vi "Open File for Writing.vi"(8 "error in (no error)":errorcluster, 11 "Configuration File in":refnum<class "Configuration File.lvclass">) -> (0 "error out":errorcluster, 1 "File was Open?":bool, 2 "refnum out":T1, 3 "Configuration File out":refnum<class "Configuration File.lvclass">)   [LabVIEW 2020, in "Configuration File.lvclass"]
doc: "The purpose of this VI is to prevent race conditions when references to files are opened in from many locations."
uses:
  Configuration File.lvclass
  C:/Git/astemes-triarc-framework/source/Framework/Configuration/Configuration.lvclass
  <vilib>/Utility/config.llb/Config Data RefNum.ctl
  Configuration/Protected/Get Config Ref.vi
  <vilib>/Utility/error.llb/Clear Errors.vi
  Base/Base.lvclass
  <vilib>/Utility/config.llb/NI_LVConfig.lvlib
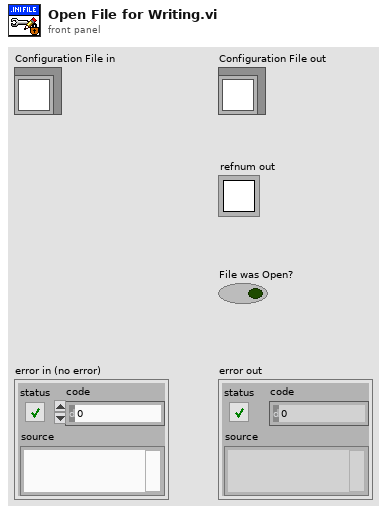
[diagram p1: front panel]
types:
  T1 = typedef "NI_LVConfig.lvlib/Config Data RefNum.ctl" = refnum<k1>
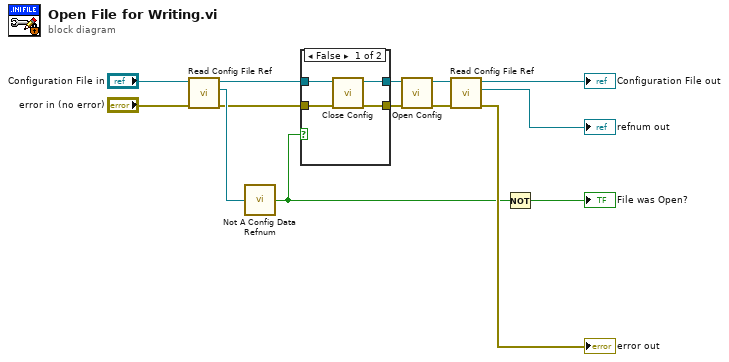
[diagram p0: block diagram]
diagram:
  n1 = call "Read Config File Ref.vi"("error in (no error)"="error in (no error)", "Configuration File In"="Configuration File in") -> ("error out"=w13:errorcluster, "refnum out"=w14:T1, "Configuration File Out"=w11:refnum<class "Configuration File.lvclass">)  [unwired: 7 in]
  n2 = call <vilib>:"Not A Config Data Refnum.vi"("refnum"=w14) -> ("not a config data refnum"=w1:bool)
  n3 = case shown="False" w1 {
    tunnel: w13 -> [w18 w19]
    tunnel: w11 -> [w17 w20]
    tunnel: [w16 w20] -> w4
    tunnel: [w15 w19] -> w3
    frame False {
      n4 = call-dynamic "Close Config.vi"("error in (no error)"=w18, "Configuration File File In"=w17) -> ("error out"=w15:errorcluster, "Configuration File File Out"=w16:refnum<class "Configuration File.lvclass">)  [unwired: 8 in]
    }
    frame True {
    }
  }
  n5 = call-dynamic "Open Config.vi"("error in (no error)"=w3, "Configuration File File In"=w4) -> ("error out"=w8:errorcluster, "Configuration File File Out"=w5:refnum<class "Configuration File.lvclass">)  [unwired: 8 in]
  n6 = call "Read Config File Ref.vi"("error in (no error)"=w8, "Configuration File In"=w5) -> ("error out"=→"error out":errorcluster, "refnum out"=→"refnum out":T1, "Configuration File Out"=→"Configuration File out":refnum<class "Configuration File.lvclass">)  [unwired: 7 in]
  n7 = Not(x=w1) -> (.not. x?=→"File was Open?":bool)
